vi "pretty.vi"(8 "error in (no error)":errorcluster, 11 "Node in":refnum<class "Node.lvclass">) -> (0 "error out":errorcluster, 2 "mlir":string, 3 "Node out":refnum<class "Node.lvclass">)   [LabVIEW 2020, in "mlir.lvlib" / "Node.lvclass"]
uses:
  Node.lvclass
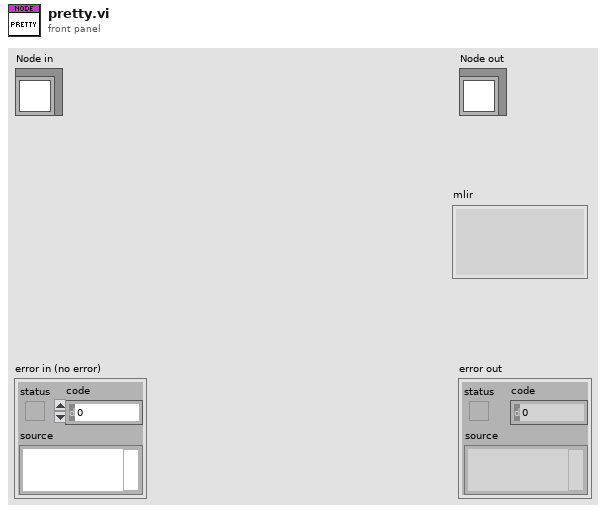
[diagram p1: front panel]
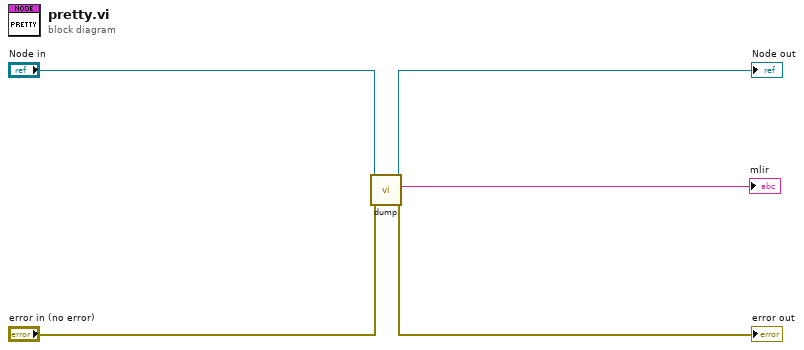
[diagram p0: block diagram]
diagram:
  n1 = call-dynamic "dump.vi"("error in (no error)"="error in (no error)", "Node in"="Node in") -> ("error out"=→"error out":errorcluster, "mlir"=→"mlir":string, "Node out"=→"Node out":refnum<class "Node.lvclass">)  [unwired: 7 in]
